vi "Target Tracker.vi"(11 "time delay":u32) -> ()   [LabVIEW 2011]
uses:
  System Set Points and States.vi
  Robot Global Data.vi
  <vilib>/addons/control/pid/pid.llb/PID (DBL).vi
  <vilib>/addons/control/pid/NI_PID_pid.lvlib
panel:
  out "Gauge":dbl(knob) scale=0.0..360.0
  out "error":dbl
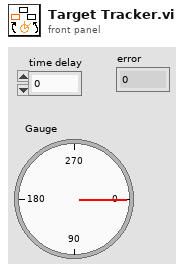
[diagram p1: front panel]
types:
  T1 = typedef "WPI_RobotDriveDevRef.ctl" = cluster{"DevStatus":errorcluster, "Motors[]":T2[], "Square Inputs":bool, "Max Output":dbl, "Isochronous":bool}
  T2 = typedef "WPI_MotorControlDeviceRef.ctl" = cluster{"DeviceStatus":errorcluster, "Type":enum16{"PWM", "CAN"}, "PWM":cluster{"Digital Module":T3, "PWM Channel":T4, "DeadBand":T5}, "CAN":cluster{"Device Number":u8, "Control Mode":T6, "Semaphore":T7, "Max Vout":dbl}, "Invert":bool, "TransformRef":T8, "InvTransformRef":T8}
  T3 = typedef "FPGA_TypedefDigitalModule.ctl" = enum16{"Digital Module 1", "Digital Module 2"}
  T4 = typedef "FPGA_DIOPWMChannel.ctl" = enum8{"PWM 1", "PWM 2", "PWM 3", "PWM 4", "PWM 5", "PWM 6", "PWM 7", "PWM 8", "PWM 9", "PWM 10", "Invalid"}
  T5 = typedef "WPI_PWMDeadband.ctl" = cluster{"Name":string, "maxPositivePwm":i32, "minPositivePwm":i32, "centerPwm":i32, "maxNegativePwm":i32, "minNegativePwm":i32, "angularRange":u16}
  T6 = typedef "WPI_CANJaguar_ControlMode.ctl" = enum8{"Percent VBus", "Current", "Speed", "Position", "Voltage"}
  T7 = typedef "Semaphore RefNum" = refnum<k1>
  T8 = typedef "WPI_PWMTransform_ConPane.ctl" = refnum<vi>
  T9 = typedef "WPI_GyroDevRef.ctl" = cluster{"DevStatus":errorcluster, "Analog Module":T10, "Analog Channel":T11, "Offset":dbl, "Gain (VoltsPerDegree/Second)":dbl}
  T10 = typedef "FPGA_TypedefAnalogModule.ctl" = enum16{"Analog Module 1", "Analog Module 2"}
  T11 = typedef "FPGA_AIChannel.ctl" = enum8{"AI 1", "AI 2", "AI 3", "AI 4", "AI 5", "AI 6", "AI 7", "AI 8", "Invalid"}
  T12 = cluster{"proportional gain (Kc)":dbl, "integral time (Ti, min)":dbl, "derivative time (Td, min)":dbl}
  T13 = cluster{"Position":cluster{"X":dbl, "Y":dbl}, "Distance (ft)":dbl}[]
  T14 = cluster{"Position":cluster{"X":dbl, "Y":dbl}, "Distance (ft)":dbl}
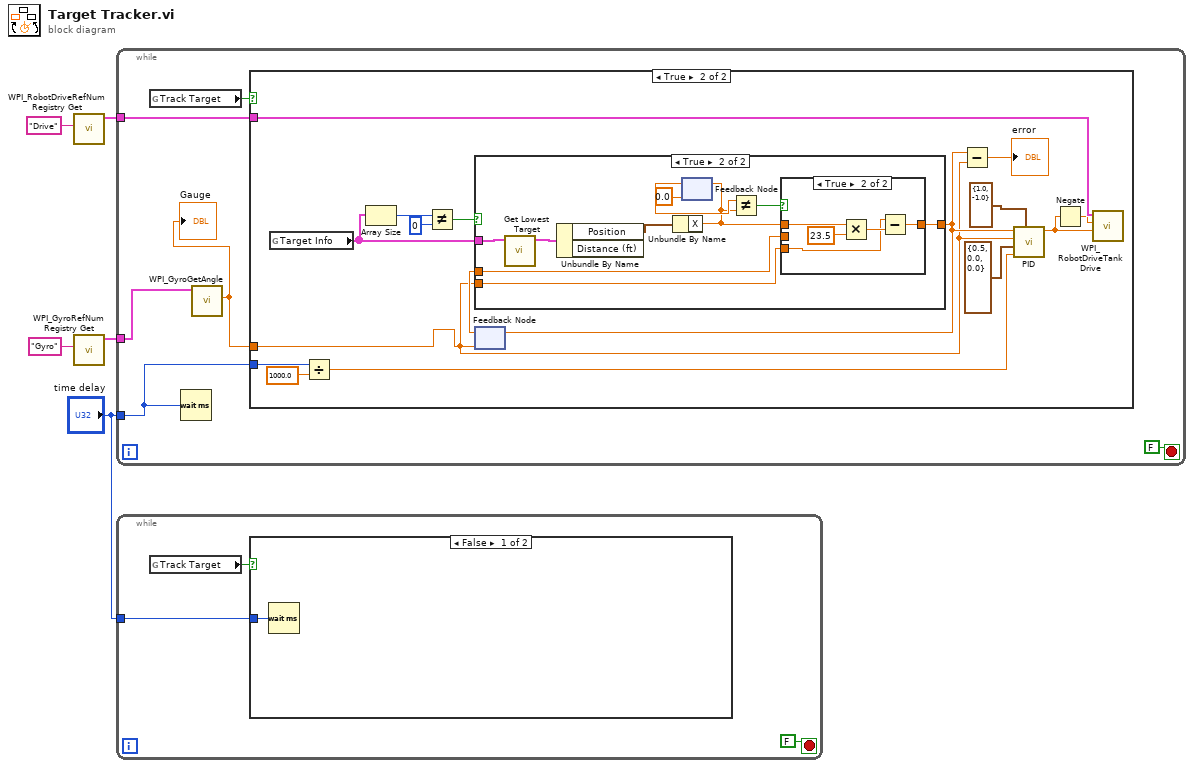
[diagram p0: block diagram]
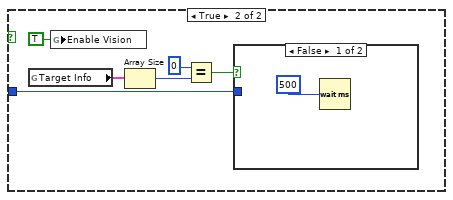
[diagram p2: hidden frame]
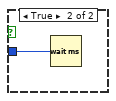
[diagram p3: hidden frame]
diagram:
  n1 = call <vilib>:"WPI_RobotDriveRefNum Registry Get.vi"("refnum name"="Drive") -> ("RobotDriveDevRef"=w2:T1)  [unwired: 9 in, 1 out]
  n2 = call <vilib>:"WPI_GyroRefNum Registry Get.vi"("refnum name"="Gyro") -> ("GyroDevRef"=w4:T9)  [unwired: 9 in, 1 out]
  n3 = while {
    tunnel: w4 -> [w7]
    tunnel: "time delay" -> [w8]
    tunnel: w2 -> [w10]
    stop <- FALSE stop-if-true
    n4 = global read "System Set Points and States.vi" "Track Target"() -> (w11:bool)
    n5 = Wait (ms)(milliseconds to wait=w8) -> ()  [unwired: 1 out]
    n6 = call <vilib>:"WPI_GyroGetAngle.vi"("GyroDevRef"=w7) -> ("Angle"=w6:dbl)  [unwired: 7 in, 3 out]
    "Gauge" <- w6
    n7 = case shown="True" w11 {
      tunnel: w10 -> [_ w27]
      tunnel: w8 -> [_ w17]
      tunnel: w6 -> [_ w12]
      frame False {
      }
      frame True {
        n8 = global read "Robot Global Data.vi" "Target Info"() -> (w22:T13)
        n9 = Divide(x=w17, y=1000.0) -> (x/y=w15:dbl)
        n10 = Array Size(array=w22) -> (size(s)=w21:i32)
        n11 = Not Equal?(x=w21, y=0) -> (x != y?=w19:bool)
        n12 = feedback #1(w12) -> (w18:dbl)
        n13 = case shown="True" w19 {
          tunnel: w22 -> [_ w34]
          tunnel: w12 -> [_ w36]
          tunnel: [w28 w35] -> w14
          tunnel: w18 -> [w28 w29]
          frame False {
          }
          frame True {
            n14 = call "Get Lowest Target.vi"("Target Info"=w34) -> ("Cluster"=w37:T14)  [unwired: 10 in]
            n15 = Unbundle By Name(w37) -> ("Position"=w38:cluster{"X":dbl, "Y":dbl})  [unwired: 1 out]
            n16 = Unbundle By Name(w38) -> ("X"=w30:dbl)
            n17 = feedback-in #2(w30) -> ()
            n18 = feedback #2(0.0 ("X")) -> (w32:dbl)
            n19 = Not Equal?(x=w32, y=w30) -> (x != y?=w31:bool)
            n20 = case shown="True" w31 {
              tunnel: w36 -> [_ w42]
              tunnel: [w39 w41] -> w35
              tunnel: w30 -> [_ w40]
              tunnel: w29 -> [w39 _]
              frame False {
              }
              frame True {
                n21 = Multiply(x=w40, y=23.5) -> (x*y=w43:dbl)
                n22 = Subtract(x=w42, y=w43) -> (x-y=w41:dbl)
              }
            }
          }
        }
        n23 = feedback-in #1(w14) -> ()
        n24 = Subtract(x=w14, y=w12) -> (x-y=→"error":dbl)
        n25 = call-poly <vilib>:"PID.vi"("output range"=cluster{"output high":dbl, "output low":dbl} {"output high"=1.0, "output low"=-1.0}, "dt (s)"=w15, "PID gains"=T12 {"proportional gain (Kc)"=0.5, "integral time (Ti, min)"=0.0, "derivative time (Td, min)"=0.0}, "process variable"=w12, "setpoint"=w14) -> ("output"=w24:dbl)  [unwired: 5 in, 1 out]
        n26 = Negate(x=w24) -> (-x=w23:dbl)
        n27 = call <vilib>:"WPI_RobotDriveTankDrive.vi"("Right axis value"=w24, "Left axis value"=w23, "RobotDriveDevRef"=w27) -> ()  [unwired: 7 in, 2 out]
      }
    }
  }
  n28 = while {
    tunnel: "time delay" -> [w46]
    stop <- FALSE stop-if-true
    n29 = global read "System Set Points and States.vi" "Track Target"() -> (w47:bool)
    n30 = case shown="False" w47 {
      tunnel: w46 -> [w48 w49]
      frame False {
        n31 = Wait (ms)(milliseconds to wait=w48) -> ()  [unwired: 1 out]
      }
      frame True {
        n32 = global read "Robot Global Data.vi" "Target Info"() -> (w54:T13)
        n33 = global write "Robot Global Data.vi" "Enable Vision"(TRUE) -> ()
        n34 = Array Size(array=w54) -> (size(s)=w52:i32)
        n35 = Equal?(x=0, y=w52) -> (x = y?=w53:bool)
        n36 = case shown="False" w53 {
          tunnel: w49 -> [_ w56]
          frame False {
            n37 = Wait (ms)(milliseconds to wait=500) -> ()  [unwired: 1 out]
          }
          frame True {
            n38 = Wait (ms)(milliseconds to wait=w56) -> ()  [unwired: 1 out]
          }
        }
      }
    }
  }
